vi "2) Temperature Conversion (F to C).vi"() -> ()   [LabVIEW 2018]
panel:
  in  "Temperature (F)":dbl(slide) scale=0.0..100.0
  out "Temperature (C)":dbl(slide) scale=0.0..100.0
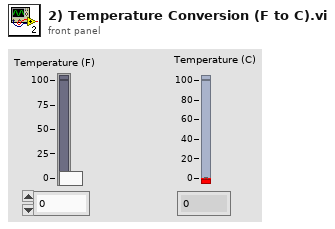
[diagram p1: front panel]
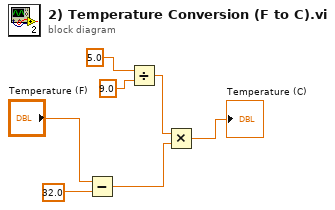
[diagram p0: block diagram]
diagram:
  n1 = Subtract(x="Temperature (F)", y=32.0 ("x-y")) -> (x-y=w6:dbl)
  n2 = Divide(x=5.0 ("x/y"), y=9.0) -> (x/y=w7:dbl)
  n3 = Multiply(x=w7, y=w6) -> (x*y=→"Temperature (C)":dbl)
